vi "remote.vi"() -> ()   [LabVIEW 2019]
uses:
  <vilib>/Utility/miscctls.llb/LVPointDoubleTypeDef.ctl
  <vilib>/Utility/miscctls.llb/LVRangeTypeDef.ctl
panel:
  in  "z0":dbl(slide) scale=-135.0..50.0
  out "Cursor.Cursor Position":T1
  in  "stop":bool
  out "XY Graph":cluster{"Horizontal":i32, "Vertical":i32}[](graph)
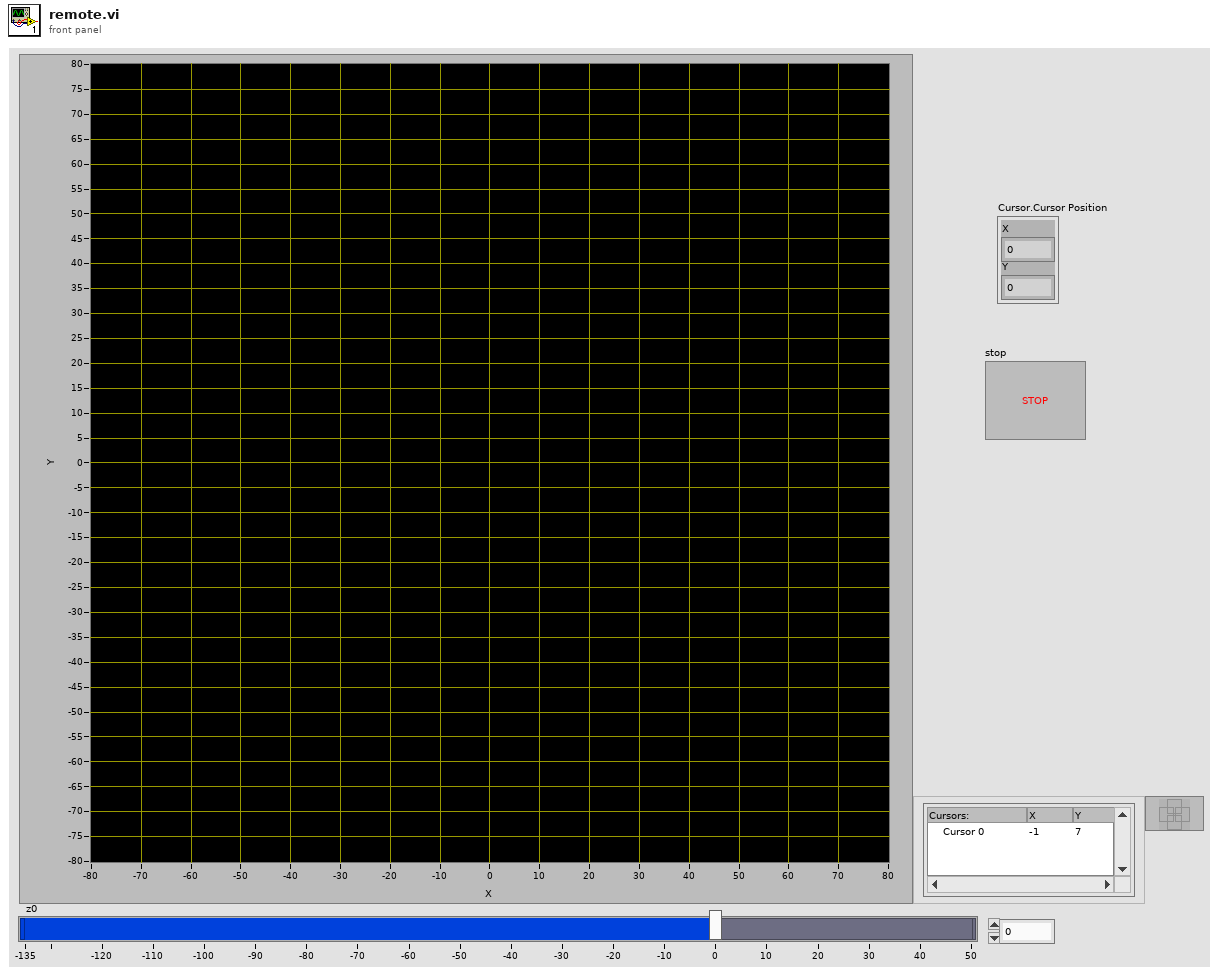
[diagram p1: front panel]
types:
  T1 = typedef "LVPointDoubleTypeDef.ctl" = cluster{"X":dbl, "Y":dbl}
  T2 = typedef "LVRangeTypeDef.ctl" = cluster{"Minimum":dbl, "Maximum":dbl, "Increment":dbl, "Minor Increment":dbl, "Start":dbl}
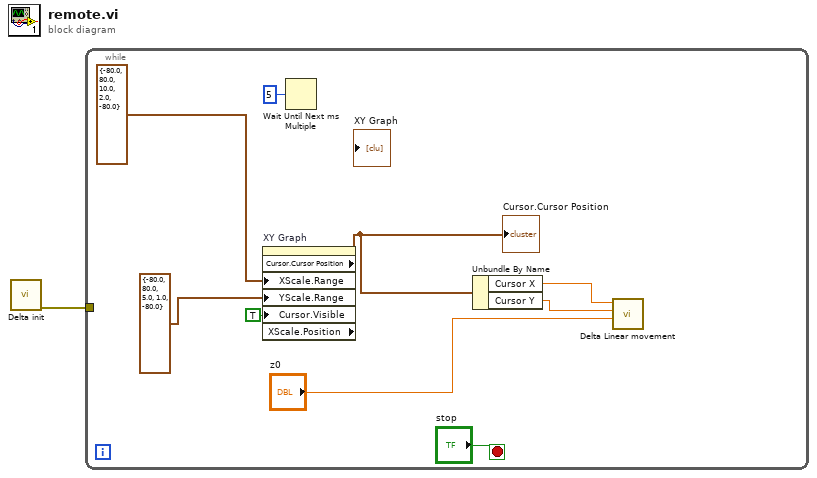
[diagram p0: block diagram]
diagram:
  n1 = call "Delta init.vi"() -> ("error out"=w1:errorcluster)  [unwired: 9 in, 2 out]
  n2 = while {
    tunnel: w1 -> [_]
    stop <- "stop" stop-if-true
    n3 = property on="XY Graph" class="XYGraph (strict)" props=["Cursor", "Cursor Position", "XScale", "Range", "YScale", "Range", "Cursor", "Visible", "XScale", "Position"]("XScale.Range"=T2 {"Minimum"=-80.0, "Maximum"=80.0, "Increment"=10.0, "Minor Increment"=2.0, "Start"=-80.0} ("X Scale.Range"), "YScale.Range"=T2 {"Minimum"=-80.0, "Maximum"=80.0, "Increment"=5.0, "Minor Increment"=1.0, "Start"=-80.0} ("Y Scale.Range"), "Cursor.Visible"=TRUE) -> ("Cursor.Cursor Position"=w4:T1)  [unwired: 2 in, 3 out]
    "Cursor.Cursor Position" <- w4
    n4 = Wait Until Next ms Multiple(millisecond multiple=u32 5) -> ()  [unwired: 1 out]
    n5 = Unbundle By Name(w4) -> ("Cursor X"=w3:dbl, "Cursor Y"=w2:dbl)
    n6 = call "Delta Linear movement.vi"("z0"="z0", "y0"=w2, "x0"=w3) -> ()  [unwired: 8 in, 1 out]
  }
